vi "Localization - Analyze and Write.vi"(11 "Select VI for Localization":path) -> (0 "error out":errorcluster)   [LabVIEW 2017, in "Localization.lvlib"]
doc: "Takes the input VI and finds all of the controls and indicators. These are then written to an Excel file with the same name along with all of the relevant information on the control or indicator. A picture of the front panel of the target VI is also saved to the Excel file so someone doing the translation can see what they are translating.\n\nChoose Movement Consulting, LLC"
uses:
  Localization.lvlib
  <vilib>/Utility/sysdir.llb/System Directory Type.ctl
  aa14743f-bee7-48c2-b079-47a9478e5ce4.vi
  <vilib>/printing/ReportDocExtensions.llb/Append Front Panel Image to Report (path).vi
  <vilib>/Utility/NIReport.llb/Append Text Table to Report (wrap).vi
  Control Info/Control Info.lvclass
  <vilib>/Utility/NIReport.llb/NI_report.lvclass
  <vilib>/Utility/NIReport.llb/NI_ReportGenerationCore.lvlib
  <vilib>/Utility/NIReport.llb/Excel/NI_Excel.lvclass
panel:
  in  "Output Directory":path
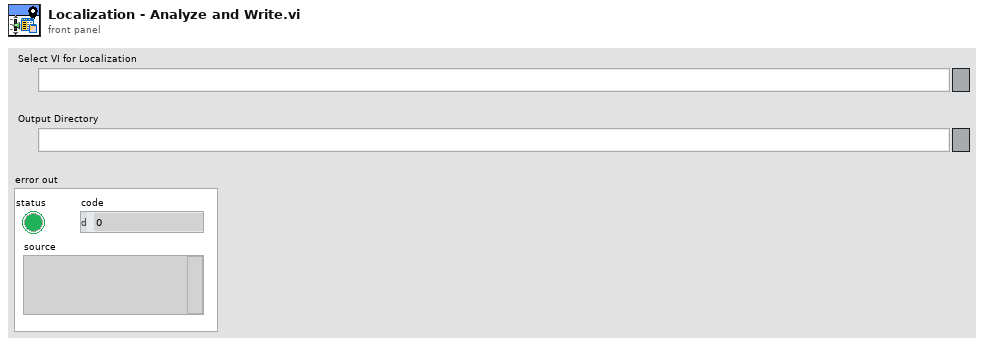
[diagram p1: front panel]
types:
  T1 = enum16{"Standard Report", "HTML", "Word", "Excel"}
  T2 = cluster{"position (excel)":cluster{"row":i32, "column":i32}, "name (excel)":string, "bookmark (word)":string}
  T3 = cluster{"on/off":bool, "weight":i32, "color":u32}
  T4 = cluster{"position (Excel)":cluster{"row":i32, "column":i32}, "name (Excel)":string, "bookmark (Word)":string}
  T5 = typedef "System Directory Type.ctl" = i32
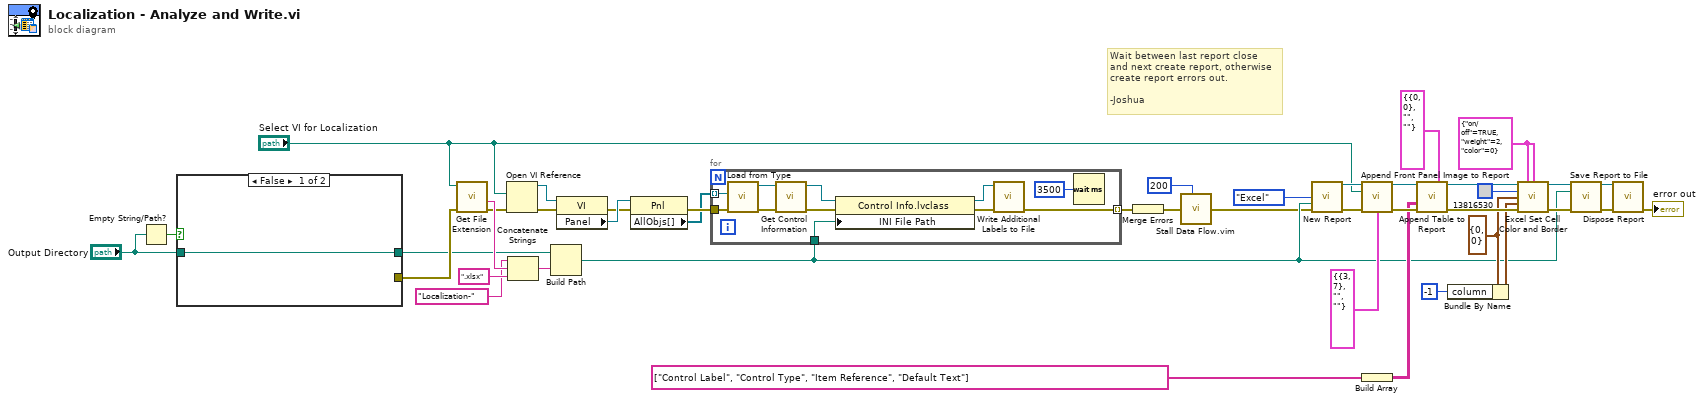
[diagram p0: block diagram]
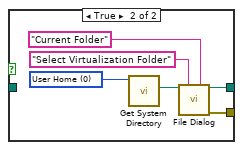
[diagram p2: hidden frame]
diagram:
  w18 = cluster{"row":i32, "column":i32} {"row"=0, "column"=0} ("start (-1, -1)")
  w26 = T3 {"on/off"=TRUE, "weight"=2, "color"=0} ("outside border")
  # "Wait between last report close\nand next create report, otherwise\ncreate report errors out.\n\n-Joshua"
  n1 = Empty String/Path?(string/path="Output Directory") -> (empty?=w6:bool)
  n2 = case shown="False" w6 {
    tunnel: [_ w45] -> w42
    tunnel: [w43 w44] -> w39
    tunnel: "Output Directory" -> [w43 _]
    frame False {
    }
    frame True {
      w48 = T5 0 items=["User Home"=0, "User Desktop"=1, "User Documents"=2, "User Application Data"=3, "User Preferences"=4, "User Temporary"=5, "Public Documents"=6, "Public Application Data"=7, "Public Preferences"=8, "Public Cache"=13, "System Core Libraries"=9, "System Installed Libraries"=10, "Application Files"=11, "Boot Volume Root"=12] ("system directory type")
      n3 = call <vilib>:"Get System Directory.vi"("system directory type"=w48) -> ("system directory"=w47:path)  [unwired: 10 in]
      n4 = call "File Dialog"("start path"=w47, "prompt"="Select Virtualization Folder", "button label"="Current Folder") -> ("selected path"=w44:path, "error out"=w45:errorcluster)  [unwired: 9 in, 2 out]
    }
  }
  n5 = call <vilib>:"Get File Extension.vi"("error in (no error)"=w42, "file"="Select VI for Localization") -> ("error out"=w37:errorcluster, "filename without extension"=w41:string)  [unwired: 5 in, 3 out]
  n6 = Open VI Reference(vi path="Select VI for Localization", error in (no error)=w37) -> (vi reference=w12:refnum<vi>, error out=w13:errorcluster)  [unwired: 4 in]
  n7 = Concatenate Strings("Localization-" ("string"), w41, ".xlsx" ("string")) -> (w38:string)
  n8 = Build Path(base path=w39, name or relative path=w38) -> (appended path=w11:path)
  n9 = property class="VI"(reference=w12, error in=w13) -> (error out=w14:errorcluster, "Panel"=w15:refnum<vi>)  [unwired: 1 out]
  n10 = property class="Pnl"(reference=w15, error in=w14) -> (error out=w10:errorcluster, "AllObjs[]"=w8:refnum<vi>[])  [unwired: 1 out]
  n11 = for {
    tunnel: w11 -> [w54]
    tunnel: w10 -> [w53]
    tunnel: [w52] -> w9 mode=indexing
    tunnel: w8 -> [w51] mode=indexing
    n12 = call "Load from Type.vi"("error in (no error)"=w53, "Control Reference"=w51) -> ("error out"=w58:errorcluster, "Control Info out"=w57:refnum<class "Control Info.lvclass">)  [unwired: 8 in]
    n13 = call-dynamic "Get Control Information.vi"("error in (no error)"=w58, "Control Info in"=w57) -> ("error out"=w55:errorcluster, "Control Info out"=w56:refnum<class "Control Info.lvclass">)  [unwired: 7 in, 1 out]
    n14 = property class="Control Info.lvclass"(reference=w56, error in=w55, "INI File Path"=w54) -> (reference out=w59:refnum<class "Control Info.lvclass">, error out=w60:errorcluster)
    n15 = call-dynamic "Write Additional Labels to File.vi"("error in (no error)"=w60, "Control Info in"=w59) -> ("error out"=w52:errorcluster)  [unwired: 8 in, 1 out]
    n16 = Wait (ms)(milliseconds to wait=u32 3500) -> ()  [unwired: 1 out]
  }
  n17 = Merge Errors(w9) -> (w4:errorcluster)
  n18 = call "Stall Data Flow.vim"("value in"=w4, "milliseconds to wait"=u32 200) -> ("value out"=w3:errorcluster)  [unwired: 1 out]
  n19 = call <vilib>:"New Report.vi"("report type"=T1."Excel", "template (empty)"=w11, "error in (no error)"=w3) -> ("report out"=w36:refnum<class "NI_report.lvclass">, "error out"=w35:errorcluster)  [unwired: 11 in]
  n20 = call-poly <vilib>:"Append Front Panel Image to Report.vi"("report in"=w36, "VI"="Select VI for Localization", "error in (no error)"=w35, "MS Office parameters"=T4 {"position (Excel)"={"row"=3, "column"=7}, "name (Excel)"="", "bookmark (Word)"=""}) -> ("report out"=w25:refnum<class "NI_report.lvclass">, "error out"=w24:errorcluster)  [unwired: 7 in, 3 out]
  n21 = Build Array(string[] ["Control Label", "Control Type", "Item Reference", "Default Text"]) -> (w22:string[][])
  n22 = call-poly <vilib>:"Append Table to Report.vi"("report in"=w25, "MS Office parameters"=T2 {"position (excel)"={"row"=0, "column"=0}, "name (excel)"="", "bookmark (word)"=""}, "text data"=w22, "error in (no error)"=w24) -> ("report out"=w29:refnum<class "NI_report.lvclass">, "error out"=w28:errorcluster)  [unwired: 8 in, 2 out]
  n23 = Bundle By Name(cluster=w18, "column"=-1) -> (w16:cluster{"row":i32, "column":i32})
  n24 = call <vilib>:"Excel Set Cell Color and Border.vi"("report in"=w29, "inside border"=w26, "outside border"=w26, "background color (w)"=u32 13816530, "start (-1, -1)"=w18, "end (-1, -1)"=w16, "error in (no error)"=w28) -> ("report out"=w20:refnum<class "NI_report.lvclass">, "error out"=w19:errorcluster)  [unwired: 7 in]
  n25 = call-dynamic "Save Report to File.vi"("report in"=w20, "report file path"=w11, "error in (no error)"=w19) -> ("report out"=w33:refnum<class "NI_report.lvclass">, "error out"=w32:errorcluster)  [unwired: 11 in]
  n26 = call-dynamic "Dispose Report.vi"("report in"=w33, "error in (no error)"=w32) -> ("error out"=→"error out":errorcluster)  [unwired: 13 in]
